vi "Main Page.vi"(8 "error in":errorcluster, 11 "Node Ptr":T2 format="%.0x") -> (0 "error out":errorcluster)   [LabVIEW 2020, in "Ballard MIL-STD-1553 System Explorer.lvlib" / "Implementation.lvlib"]
uses:
  Implementation.lvlib
  <vilib>/NI VeriStand/Custom Device API/Custom Device Item Ref.ctl
  Shared/Initialization Method.ctl
  <vilib>/NI VeriStand/Custom Device API/Custom Device API.lvlib
  Scripting/Ballard MIL-STD-1553 Scripting.lvlib
panel:
  in  "core number":i32 caption="Core Number" min=0 step=1
  in  "number":i32=1 caption="PXI Slot Number" min=0 step=1
  in  "initialization method":T1 caption="Initialization Method"
  out "Version":string
  in  "SHDocVw.IWebBrowser":refnum<k7>(container)
  in  "General Header":cluster{"Section Name":string}={"Section Name"="Ballard MIL-STD-1553 - Main"}
  in  "Description":string
  in  "Name":string
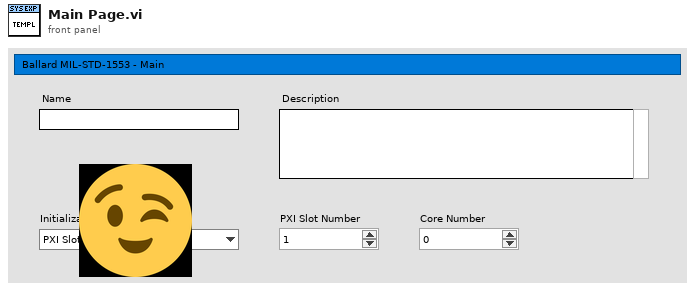
[diagram p1: front panel]
types:
  T1 = typedef "Initialization Method.ctl" = enum16{"PXI Slot Number", "Card Number"}
  T2 = typedef "Custom Device API.lvlib/Custom Device Item Ref.ctl" = u64
  T3 = typedef "Device Parameters.ctl" = cluster{"initialization method":T1, "card number":i32, "PXI slot number":i32, "core number":i32}
  T4 = typedef "Custom Device API.lvlib/Custom Device Item Info.ctl" = cluster{"Name":string, "Is Channel":bool, "GUID":string, "Is Waveform":bool}
  T5 = typedef "Custom Device API.lvlib/Custom Device Commands.ctl" = enum16{"Default", "Item renamed", "Shutdown", "Dynamic button pressed"}
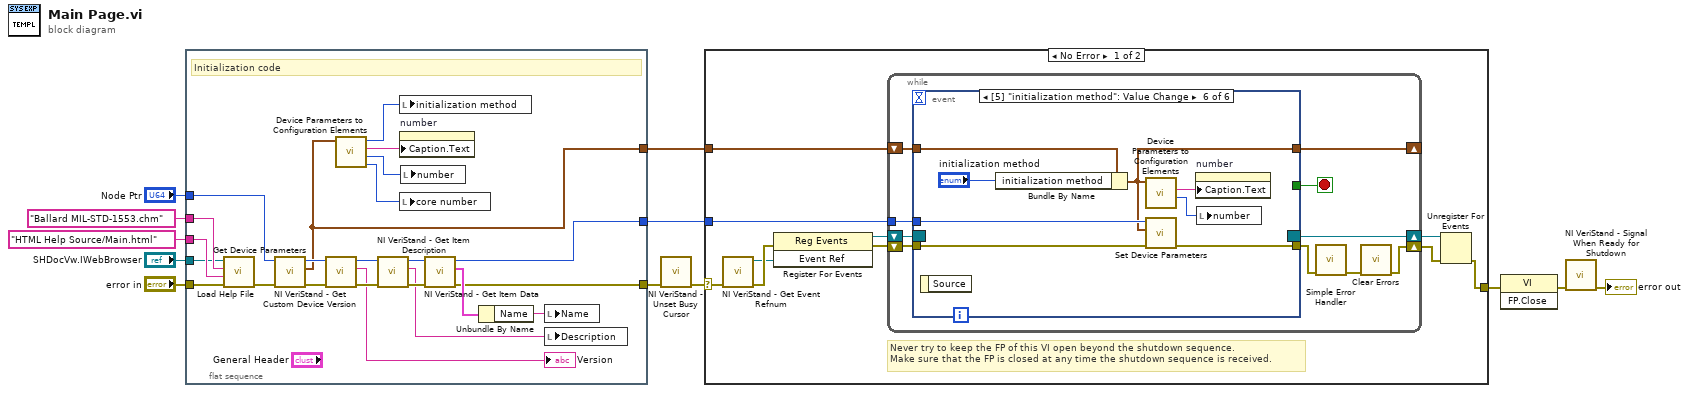
[diagram p0: block diagram]
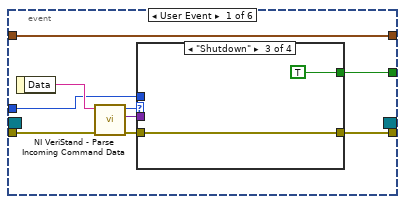
[diagram p2: hidden frame]
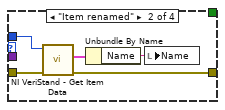
[diagram p4: hidden frame]
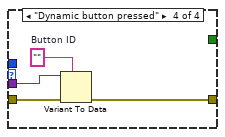
[diagram p5: hidden frame]
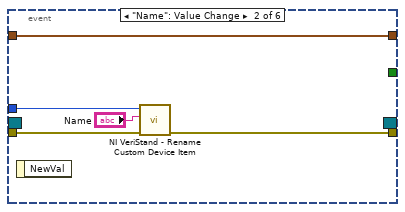
[diagram p6: hidden frame]
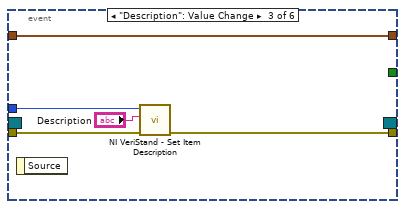
[diagram p7: hidden frame]
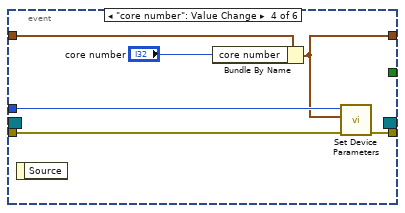
[diagram p8: hidden frame]
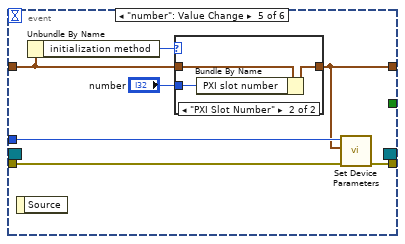
[diagram p9: hidden frame]
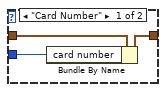
[diagram p10: hidden frame]
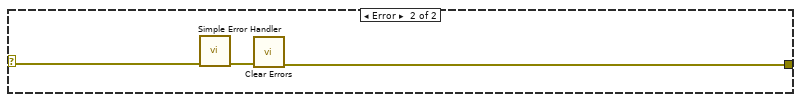
[diagram p11: hidden frame]
diagram:
  n1 = flat-sequence "Initialization code" {
    tunnel: "error in" -> [w27]
    tunnel: "Node Ptr" -> [w22]
    tunnel: [w17] -> w8
    tunnel: [w18] -> w5
    tunnel: "SHDocVw.IWebBrowser" -> [w24]
    tunnel: "HTML Help Source/Main.html" ("HTML File") -> [w25]
    tunnel: "Ballard MIL-STD-1553.chm" ("CD_CHM_FileName") -> [w26]
    tunnel: [w13] -> w1
    frame #0 {
      # "Initialization code"
      n2 = call "Load Help File.vi"("error in (no error)"=w27, "HTML File to Load"=w25, "Main CHM File"=w26, "Browser"=w24) -> ("error out"=w21:errorcluster)  [unwired: 7 in]
      n3 = call "Get Device Parameters.vi"("error in"=w21, "Ballard MIL-STD 1553 custom device in"=w22) -> ("error out"=w20:errorcluster, "device parameters"=w13:T3, "Ballard MIL-STD 1553 custom device out"=w19:T2)  [unwired: 7 in]
      n4 = call <vilib>:"NI VeriStand - Get Custom Device Version.vi"("error in (no error)"=w20, "Device Ref in"=w19) -> ("error out"=w32:errorcluster, "Value"=→"Version":string, "Device Ref out"=w31:T2)  [unwired: 7 in]
      n5 = call "Device Parameters to Configuration Elements.vi"("device parameters"=w13) -> ("core number"=w14:i32, "number"=w15:i32, "number caption"=w16:string, "initialization method"=w23:T1)  [unwired: 7 in]
      n6 = call <vilib>:"NI VeriStand - Get Item Description.vi"("error in (no error)"=w32, "Item Ref in"=w31) -> ("error out"=w34:errorcluster, "Description"=w28:string, "Item Ref out"=w35:T2)  [unwired: 7 out]
      n7 = local write "initialization method"(w23) -> ()
      n8 = property on="number" class="DigNum (strict)"("Caption.Text"=w16) -> ()  [unwired: 2 in, 2 out]
      n9 = local write "core number"(w14) -> ()
      n10 = local write "number"(w15) -> ()
      n11 = call <vilib>:"NI VeriStand - Get Item Data.vi"("error in (no error)"=w34, "Item Ref in"=w35) -> ("error out"=w17:errorcluster, "Item Info"=w33:T4, "Item Ref out"=w18:T2)  [unwired: 7 out]
      n12 = Unbundle By Name(w33) -> ("Name"=w29:string)
      n13 = local write "Name"(w29) -> ()
      n14 = local write "Description"(w28) -> ()
    }
  }
  n15 = call <vilib>:"NI VeriStand - Unset Busy Cursor.vi"("error in (no error)"=w8) -> ("error out"=w7:errorcluster)  [unwired: 10 out]
  n16 = case shown="No Error" w7 {
    selector: w7 -> [w37 w116]
    tunnel: [w42 w114] -> w12
    tunnel: w5 -> [w38 _]
    tunnel: w1 -> [w36 _]
    frame No Error {
      # "Never try to keep the FP of this VI open beyond the shutdown sequence.\nMake sure that the FP is closed at any time the shutdown sequence is received."
      n17 = call <vilib>:"NI VeriStand - Get Event Refnum.vi"("error in (no error)"=w37) -> ("error out"=w45:errorcluster, "Event Ref"=w41:refnum<user-event>)  [unwired: 9 out]
      n18 = register-events(error in=w45, w41) -> (reference out=w39:refnum<event-registration>, error out=w40:errorcluster)  [unwired: 1 in]
      n19 = while {
        tunnel: w38 -> [w51]
        shift-right: [w48] -> w43
        shift-left: w40 -> [w54]
        shift-right: [w55] -> w44
        shift-left: w39 -> [w53]
        shift-right: [w46] -> _
        shift-left: w36 -> [w47]
        stop <- w52 stop-if-true
        n20 = event shown="[5] \"initialization method\": Value Change" {
          selector: w53 -> [_ _ _ _ _ _]
          dyn-events: [_ _ _ _ _ _] -> w55
          timeout: _ -> [_ _ _ _ _ _]
          tunnel: w54 -> [w64 w81 w85 w88 w96 w107]
          tunnel: [w60 _ _ _ _ _] -> w52
          tunnel: [w59 w80 w84 w89 w95 w106] -> w50
          tunnel: w51 -> [w56 w79 w86 w90 w94 w109]
          tunnel: w47 -> [w57 w77 w82 w92 w98 w111]
          tunnel: [w57 w77 w82 w87 w93 w108] -> w46
          event User Event {
            n21 = event-data() -> ("Data"=w63:string)  [unwired: 1 out]
            n22 = call <vilib>:"NI VeriStand - Parse Incoming Command Data.vi"("error in (no error)"=w64, "Incoming data"=w63) -> ("error out"=w62:errorcluster, "Outgoing data"=w58:variant, "Action"=w61:T5)  [unwired: 7 out]
            n23 = case shown="\"Shutdown\"" w61 {
              tunnel: w62 -> [w65 w70 w71 w76]
              tunnel: [_ _ TRUE _] -> w60
              tunnel: [w65 w67 w71 w73] -> w59
              tunnel: w56 -> [_ w69 _ _]
              tunnel: w58 -> [_ _ _ w75]
              frame "Default", Default {
              }
              frame "Item renamed" {
                n24 = call <vilib>:"NI VeriStand - Get Item Data.vi"("error in (no error)"=w70, "Item Ref in"=w69) -> ("error out"=w67:errorcluster, "Item Info"=w68:T4)  [unwired: 8 out]
                n25 = Unbundle By Name(w68) -> ("Name"=w66:string)
                n26 = local write "Name"(w66) -> ()
              }
              frame "Shutdown" {
              }
              frame "Dynamic button pressed" {
                w74 = ""  # Button ID
                n27 = Variant To Data(error in=w76, type=w74, Variant=w75) -> (error out=w73:errorcluster)  [unwired: 1 out]
              }
            }
          }
          event "Name": Value Change {
            n28 = event-data() -> ()  [unwired: 2 out]
            n29 = call <vilib>:"NI VeriStand - Rename Custom Device Item.vi"("error in (no error)"=w81, "New Name"="Name", "Item Ref in"=w79) -> ("error out"=w80:errorcluster)  [unwired: 1 in, 7 out]
          }
          event "Description": Value Change {
            n30 = event-data() -> ()  [unwired: 2 out]
            n31 = call <vilib>:"NI VeriStand - Set Item Description.vi"("error in (no error)"=w85, "Description"="Description", "Item Ref in"=w86) -> ("error out"=w84:errorcluster)  [unwired: 8 out]
          }
          event "core number": Value Change {
            n32 = event-data() -> ()  [unwired: 2 out]
            n33 = Bundle By Name(cluster=w92, "core number"="core number") -> (w87:T3)
            n34 = call "Set Device Parameters.vi"("error in"=w88, "device parameters"=w87, "Ballard MIL-STD 1553 custom device in"=w90) -> ("error out"=w89:errorcluster)  [unwired: 7 in, 1 out]
          }
          event "number": Value Change {
            n35 = event-data() -> ()  [unwired: 2 out]
            n36 = Unbundle By Name(w98) -> ("initialization method"=w99:T1)
            n37 = case shown="\"PXI Slot Number\"" w99 {
              tunnel: w98 -> [w102 w105]
              tunnel: "number" -> [w101 w104]
              tunnel: [w100 w103] -> w93
              frame "Card Number" {
                n38 = Bundle By Name(cluster=w102, "card number"=w101) -> (w100:T3)
              }
              frame "PXI Slot Number" {
                n39 = Bundle By Name(cluster=w105, "PXI slot number"=w104) -> (w103:T3)
              }
            }
            n40 = call "Set Device Parameters.vi"("error in"=w96, "device parameters"=w93, "Ballard MIL-STD 1553 custom device in"=w94) -> ("error out"=w95:errorcluster)  [unwired: 7 in, 1 out]
          }
          event Value Change {
            n41 = event-data() -> ()  [unwired: 2 out]
            n42 = Bundle By Name(cluster=w111, "initialization method"="initialization method") -> (w108:T3)
            n43 = call "Device Parameters to Configuration Elements.vi"("device parameters"=w108) -> ("number"=w112:i32, "number caption"=w113:string)  [unwired: 7 in, 2 out]
            n44 = call "Set Device Parameters.vi"("error in"=w107, "device parameters"=w108, "Ballard MIL-STD 1553 custom device in"=w109) -> ("error out"=w106:errorcluster)  [unwired: 7 in, 1 out]
            n45 = property on="number" class="DigNum (strict)"("Caption.Text"=w113) -> ()  [unwired: 2 in, 2 out]
            n46 = local write "number"(w112) -> ()
          }
        }
        n47 = call <vilib>:"Simple Error Handler.vi"("error in (no error)"=w50) -> ("error out"=w49:errorcluster)  [unwired: 1 in, 7 out]
        n48 = call <vilib>:"Clear Errors.vi"("error in (no error)"=w49) -> ("error out"=w48:errorcluster)  [unwired: 1 in, 5 out]
      }
      n49 = Unregister For Events(event registration refnum=w44, error in=w43) -> (error out=w42:errorcluster)
    }
    frame Error {
      n50 = call <vilib>:"Simple Error Handler.vi"("error in (no error)"=w116) -> ("error out"=w115:errorcluster)  [unwired: 1 in, 7 out]
      n51 = call <vilib>:"Clear Errors.vi"("error in (no error)"=w115) -> ("error out"=w114:errorcluster)  [unwired: 1 in, 5 out]
    }
  }
  n52 = invoke class="VI" method="FP.Close"(error in=w12) -> (error out=w11:errorcluster)  [unwired: 2 in, 2 out]
  n53 = call <vilib>:"NI VeriStand - Signal When Ready for Shutdown.vi"("error in (no error)"=w11) -> ("error out"=→"error out":errorcluster)  [unwired: 10 out]
